vi "1 - 测试基台交互.vi"(6 "测试机台选择":tag="VB8012-30F490B", 8 "逻辑分析仪参数输入":T2, 9 "可编程电源参数输入":T3, 10 "显示控件引用输入":T1) -> (0 "error out":errorcluster caption="错误输出", 2 "采集信号输出":waveform(dbl)[](array[waveform]), 3 "显示控件引用输出":T1)   [LabVIEW 2019]
uses:
  <vilib>/VirtualBench/_PS Configure Voltage Output0.vi
  <vilib>/VirtualBench/_FGEN Configure Standard Waveform14.vi
  <vilib>/VirtualBench/_MSO Configure Timing0.vi
  <vilib>/VirtualBench/_MSO Configure Digital Edge Trigger0.vi
  <vilib>/VirtualBench/_MSO Configure Analog Edge Trigger0.vi
  <vilib>/VirtualBench/_MSO Configure Digital Pattern Trigger0.vi
  <vilib>/VirtualBench/_FGEN Configure Standard Waveform0.vi
  <vilib>/VirtualBench/VirtualBench.lvlib
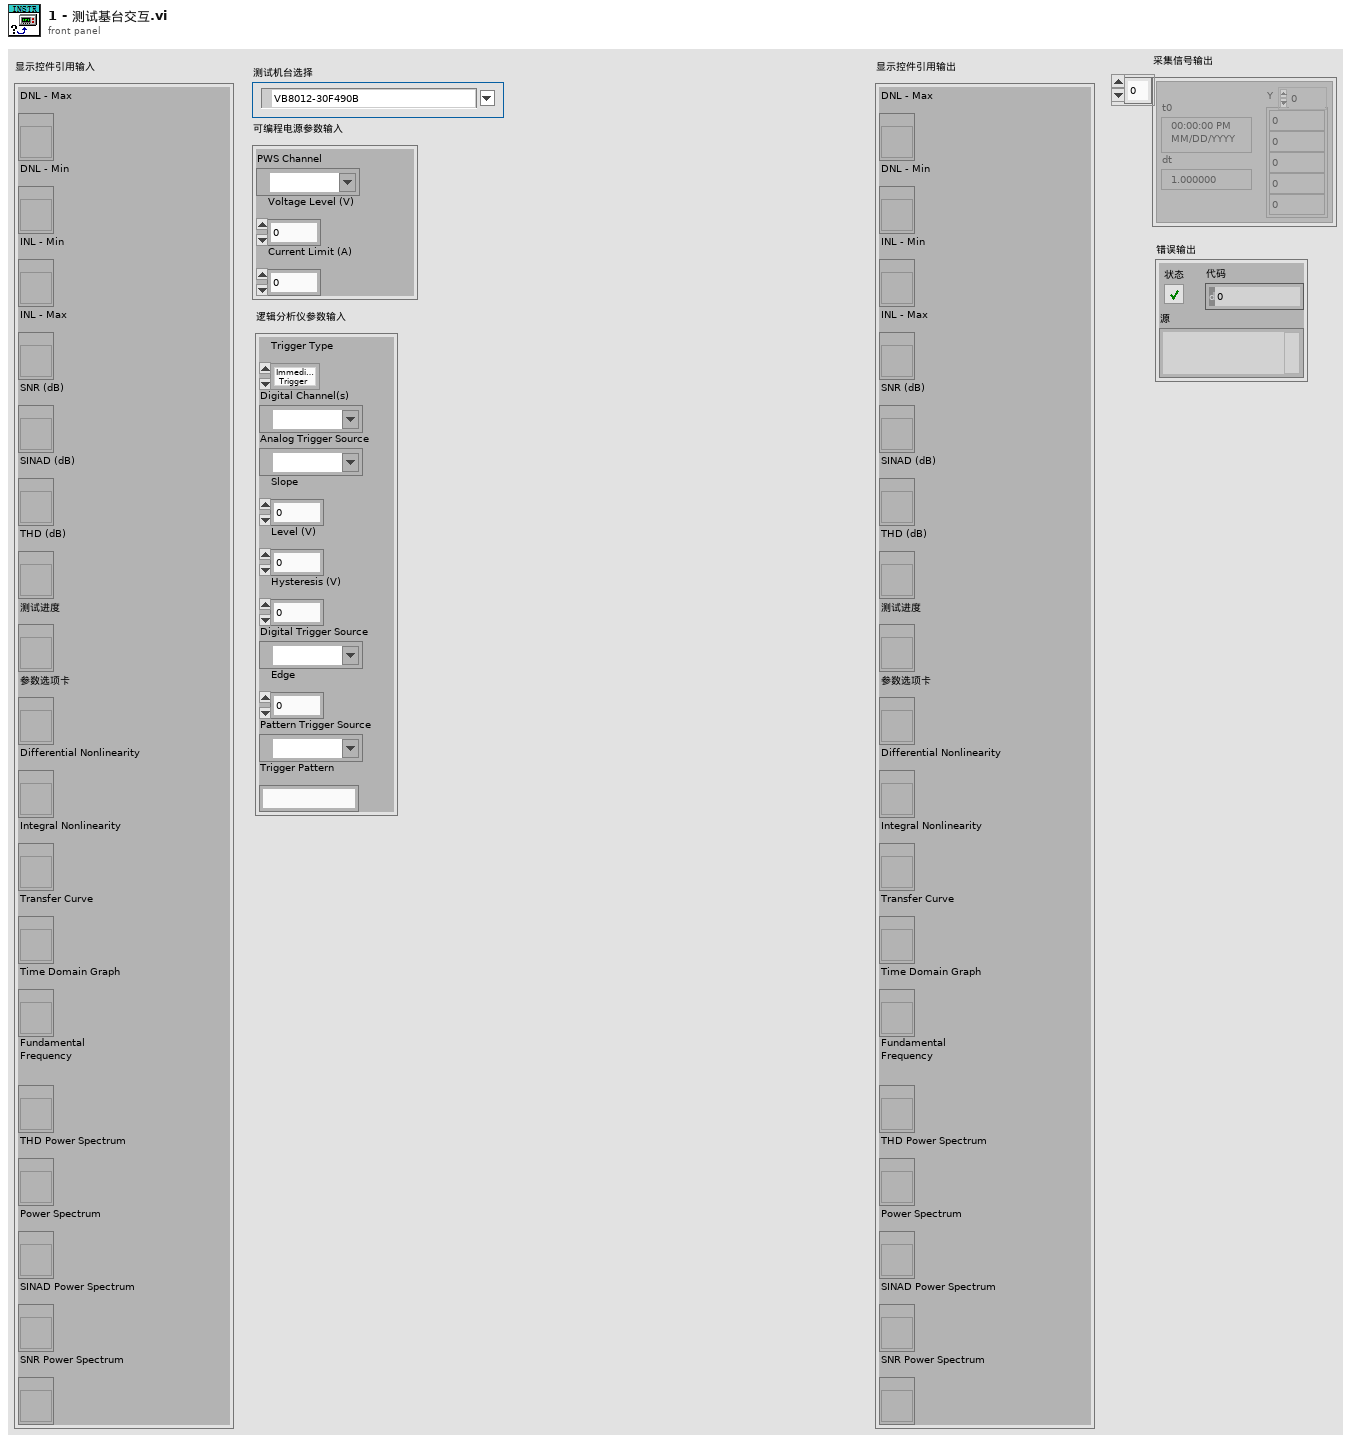
[diagram p1: front panel]
types:
  T1 = cluster{"DNL - Max":refnum<vi>, "DNL - Min":refnum<vi>, "INL - Min":refnum<vi>, "INL - Max":refnum<vi>, "SNR (dB)":refnum<vi>, "SINAD (dB)":refnum<vi>, "THD (dB)":refnum<vi>, "测试进度":refnum<vi>, "参数选项卡":refnum<vi>, "Differential Nonlinearity":refnum<vi>, "Integral Nonlinearity":refnum<vi>, "Transfer Curve":refnum<vi>, "Time Domain Graph":refnum<vi>, "Fundamental\nFrequency":refnum<vi>, "THD Power Spectrum":refnum<vi>, "Power Spectrum":refnum<vi>, "SINAD Power Spectrum":refnum<vi>, "SNR Power Spectrum":refnum<vi>}
  T2 = cluster{"Trigger Type":enum32{"Immediate Trigger", "Digital Trigger", "Analog Trigger", "Pattern Trigger"}, "Digital Channel(s)":tag, "Analog Trigger Source":tag, "Slope":i32, "Level (V)":dbl, "Hysteresis (V)":dbl, "Digital Trigger Source":tag, "Edge":i32, "Pattern Trigger Source":tag, "Trigger Pattern":string}
  T3 = cluster{"PWS Channel":tag, "Voltage Level (V)":dbl, "Current Limit (A)":dbl}
  T4 = enum32{"Time Domain", "Power Spectrum", "THD", "SINAD", "SNR", "DNL", "INL", "Transfer Curve"}
  T5 = enum32{"Immediate Trigger", "Digital Trigger", "Analog Trigger", "Pattern Trigger"}
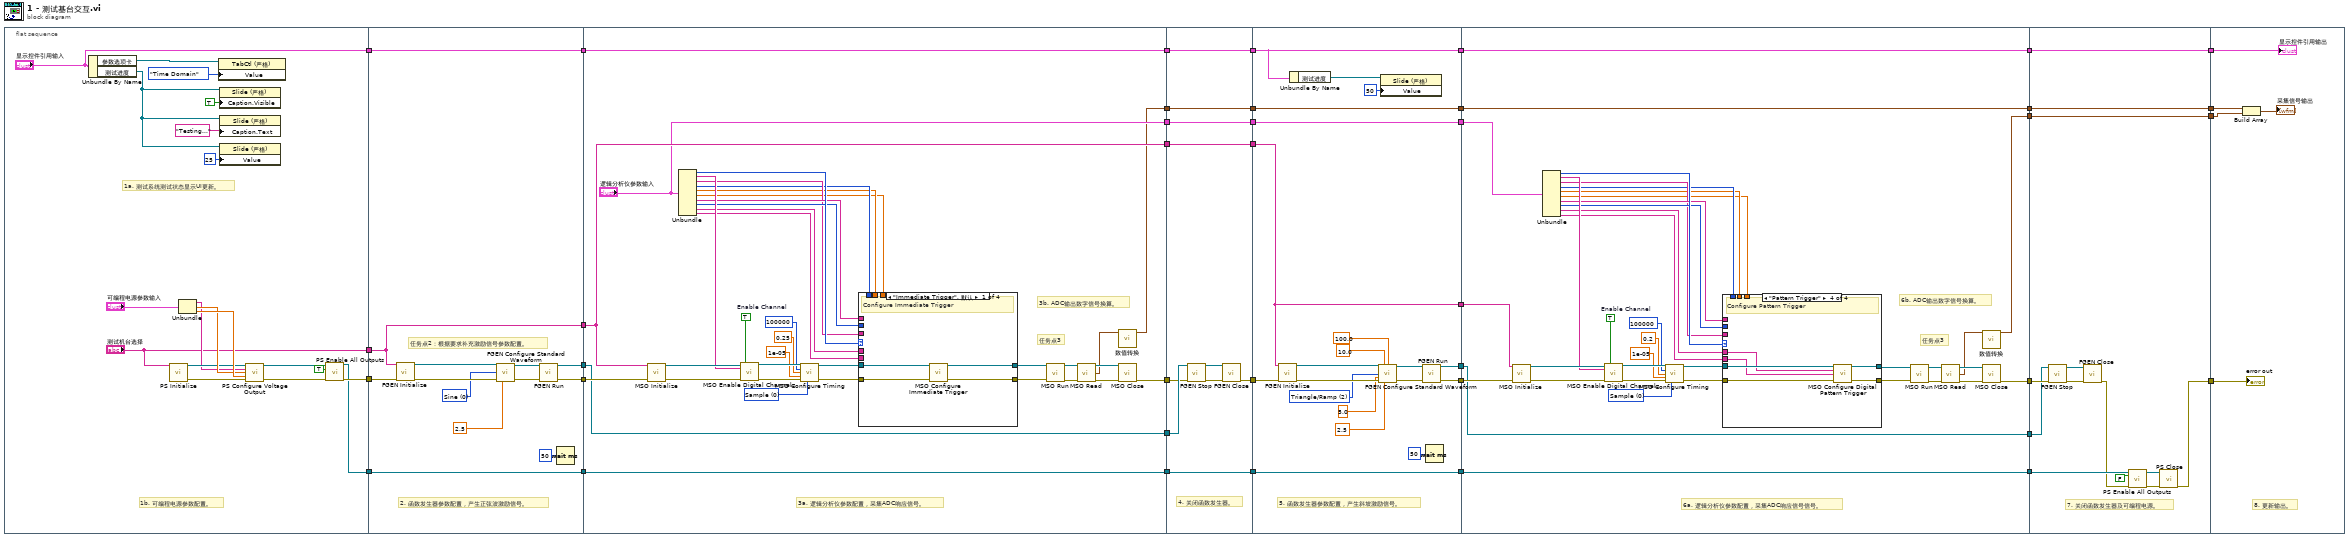
[diagram p0: block diagram]
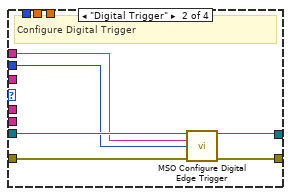
[diagram p2: hidden frame]
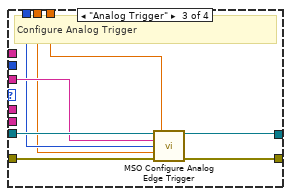
[diagram p3: hidden frame]
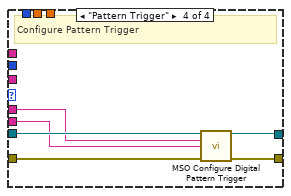
[diagram p4: hidden frame]
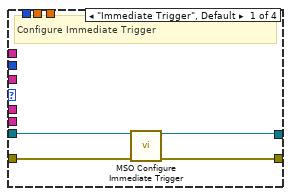
[diagram p5: hidden frame]
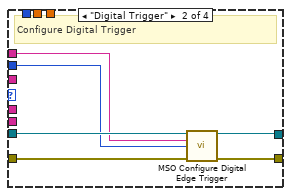
[diagram p6: hidden frame]
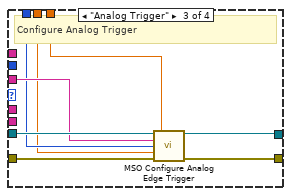
[diagram p7: hidden frame]
diagram:
  n1 = flat-sequence {
    tunnel: [w49] -> w39
    tunnel: ["测试机台选择"] -> w38
    tunnel: ["显示控件引用输入"] -> w8
    tunnel: [w47] -> w6
    tunnel: w39 -> [w67]
    tunnel: w38 -> [w62]
    tunnel: [w64] -> w37
    tunnel: [w63] -> w36
    tunnel: [w62] -> w35
    tunnel: [w61] -> w9
    tunnel: w8 -> [w61]
    tunnel: w6 -> [w60]
    tunnel: [w60] -> w1
    tunnel: w37 -> [w78]
    tunnel: w36 -> [w95]
    tunnel: w35 -> [w76]
    tunnel: [w78] -> w34
    tunnel: [w77] -> w33
    tunnel: [w76] -> w30
    tunnel: ["逻辑分析仪参数输入"] -> w25
    tunnel: [w74] -> w21
    tunnel: [w73] -> w10
    tunnel: w9 -> [w73]
    tunnel: [w72] -> w2
    tunnel: w1 -> [w72]
    tunnel: w34 -> [w140]
    tunnel: w33 -> [w139]
    tunnel: [w137] -> w32
    tunnel: [w136] -> w31
    tunnel: w30 -> [w136]
    tunnel: [w135] -> w26
    tunnel: w25 -> [w135]
    tunnel: w21 -> [w134]
    tunnel: [w134] -> w18
    tunnel: [w133] -> w11
    tunnel: w10 -> [w133]
    tunnel: [w132] -> w3
    tunnel: w2 -> [w132]
    tunnel: w32 -> [w152]
    tunnel: w31 -> [w149]
    tunnel: [w151] -> w29
    tunnel: [w150] -> w28
    tunnel: [w149] -> w27
    tunnel: w26 -> [w148]
    tunnel: [w148] -> w24
    tunnel: [w147] -> w19
    tunnel: w18 -> [w147]
    tunnel: [w142] -> w12
    tunnel: w11 -> [w142]
    tunnel: [w146] -> w4
    tunnel: w3 -> [w146]
    tunnel: w29 -> [w171]
    tunnel: w28 -> [w167]
    tunnel: w27 -> [w170]
    tunnel: w24 -> [w169]
    tunnel: [w168] -> w23
    tunnel: [w167] -> w22
    tunnel: [w166] -> w20
    tunnel: w19 -> [w166]
    tunnel: [w163] -> w17
    tunnel: [w165] -> w13
    tunnel: w12 -> [w165]
    tunnel: [w164] -> w5
    tunnel: w4 -> [w164]
    tunnel: w23 -> [w233]
    tunnel: w22 -> [w232]
    tunnel: w20 -> [w231]
    tunnel: w17 -> [w230]
    tunnel: [w231] -> w16
    tunnel: [w230] -> w15
    tunnel: [w229] -> w14
    tunnel: w13 -> [w229]
    tunnel: [w223] -> w7
    tunnel: w5 -> [w225]
    tunnel: w16 -> [w240]
    tunnel: w15 -> [w239]
    tunnel: w14 -> [w236]
    tunnel: w7 -> [w237]
    frame #0 {
      # "1b. 可编程电源参数配置。"
      # "1a. 测试系统测试状态显示UI更新。"
      n2 = Unbundle By Name("显示控件引用输入") -> ("参数选项卡"=w46:refnum<vi>, "测试进度"=w42:refnum<vi>)
      n3 = call <vilib>:"PS Initialize.vi"("Device Name"="测试机台选择") -> ("Instrument Handle Out"=w55:refnum<k21>, "Error Out"=w51:errorcluster)  [unwired: 13 in]
      n4 = Unbundle("可编程电源参数输入") -> ("PWS Channel"=w54:tag, "Voltage Level (V)"=w56:dbl, "Current Limit (A)"=w57:dbl)
      n5 = property class="TabCtl (严格)"(reference=w46, "Value"=T4."Time Domain" ("值")) -> ()  [unwired: 1 in, 2 out]
      n6 = property class="Slide (严格)"(reference=w42, "Caption.Visible"=TRUE ("标题.可见")) -> ()  [unwired: 1 in, 2 out]
      n7 = property class="Slide (严格)"(reference=w42, "Caption.Text"="Testing..." ("标题.文本")) -> ()  [unwired: 1 in, 2 out]
      n8 = property class="Slide (严格)"(reference=w42, "Value"=u8 25 ("值")) -> ()  [unwired: 1 in, 2 out]
      n9 = call-poly <vilib>:"PS Configure Voltage Output.vi"("Instrument Handle In"=w55, "Channel"=w54, "Voltage Level"=w56, "Current Limit"=w57, "Error In"=w51) -> ("Instrument Handle Out"=w58:refnum<k21>, "Error Out"=w52:errorcluster)  [unwired: 9 in]
      n10 = call <vilib>:"PS Enable All Outputs.vi"("Instrument Handle In"=w58, "Enable Outputs"=TRUE ("Enable Output"), "Error In"=w52) -> ("Instrument Handle Out"=w47:refnum<k21>, "Error Out"=w49:errorcluster)  [unwired: 11 in]
    }
    frame #1 {
      w66 = 0 items=["Sine", "Square", "Triangle/Ramp", "DC"] ("Waveform Function")
      # "任务点2：根据要求补充激励信号参数配置。"
      # "2. 函数发生器参数配置，产生正弦波激励信号。"
      n11 = call <vilib>:"FGEN Initialize.vi"("Device Name"=w62, "Error In"=w67) -> ("Instrument Handle Out"=w68:refnum<k21>, "Error Out"=w69:errorcluster)  [unwired: 12 in]
      n12 = call-poly <vilib>:"FGEN Configure Standard Waveform.vi"("Instrument Handle In"=w68, "Waveform Function"=w66, "Error In"=w69, "DC Offset"=2.5 ("DC Offset (V)")) -> ("Instrument Handle Out"=w70:refnum<k21>, "Error Out"=w71:errorcluster)  [unwired: 10 in]
      n13 = call <vilib>:"FGEN Run.vi"("Instrument Handle In"=w70, "Error In"=w71) -> ("Instrument Handle Out"=w64:refnum<k21>, "Error Out"=w63:errorcluster)  [unwired: 12 in]
      n14 = Wait (ms)(milliseconds to wait=u32 50 ("等待时间（毫秒）")) -> ()  [unwired: 1 out]
    }
    frame #2 {
      w102 = TRUE  # Enable Channel
      w107 = 0 items=["Sample", "Peak Detect"] ("Sampling Mode")
      # "任务点3"
      # "3b. ADC输出数字信号换算。"
      # "3a. 逻辑分析仪参数配置，采集ADC响应信号。"
      n15 = call <vilib>:"MSO Initialize.vi"("Device Name"=w76, "Error In"=w95) -> ("Instrument Handle Out"=w99:refnum<k21>, "Error Out"=w98:errorcluster)  [unwired: 12 in]
      n16 = Unbundle("逻辑分析仪参数输入") -> ("Trigger Type"=w90:T5, "Digital Channel(s)"=w94:tag, "Analog Trigger Source"=w87:tag, "Slope"=w86:i32, "Level (V)"=w85:dbl, "Hysteresis (V)"=w84:dbl, "Digital Trigger Source"=w89:tag, "Edge"=w88:i32, "Pattern Trigger Source"=w83:tag, "Trigger Pattern"=w82:string)
      n17 = call <vilib>:"MSO Enable Digital Channels.vi"("Instrument Handle In"=w99, "Enable Channel"=w102, "Channel"=w94, "Error In"=w98) -> ("Instrument Handle Out"=w103:refnum<k21>, "Error Out"=w104:errorcluster)  [unwired: 10 in]
      n18 = call-poly <vilib>:"MSO Configure Timing.vi"("Instrument Handle In"=w103, "Sample Rate"=100000 ("Sample Rate (Hz)"), "Acquisition Time (s)"=0.25, "Pretrigger Time (s)"=1e-05, "Error In"=w104, "Sampling Mode"=w107) -> ("Instrument Handle Out"=w106:refnum<k21>, "Error Out"=w105:errorcluster)  [unwired: 8 in]
      n19 = case shown="\"Immediate Trigger\", 默认" w90 {
        tunnel: w106 -> [w111 w115 w122 w129]
        tunnel: w105 -> [w109 w116 w125 w128]
        tunnel: [w110 w114 w123 w130] -> w97
        tunnel: [w108 w117 w124 w131] -> w96
        tunnel: w89 -> [_ w113 _ _]
        tunnel: w88 -> [_ w112 _ _]
        tunnel: w87 -> [_ _ w121 _]
        tunnel: w86 -> [_ _ w120 _]
        tunnel: w85 -> [_ _ w119 _]
        tunnel: w84 -> [_ _ w118 _]
        tunnel: w83 -> [_ _ _ w127]
        tunnel: w82 -> [_ _ _ w126]
        frame "Immediate Trigger", Default {
          # "Configure Immediate Trigger"
          n20 = call <vilib>:"MSO Configure Immediate Trigger.vi"("Instrument Handle In"=w111, "Error In"=w109) -> ("Instrument Handle Out"=w110:refnum<k21>, "Error Out"=w108:errorcluster)  [unwired: 12 in]
        }
        frame "Digital Trigger" {
          # "Configure Digital Trigger"
          n21 = call-poly <vilib>:"MSO Configure Digital Edge Trigger.vi"("Instrument Handle In"=w115, "Trigger Source"=w113, "Trigger Slope"=w112, "Error In"=w116) -> ("Instrument Handle Out"=w114:refnum<k21>, "Error Out"=w117:errorcluster)  [unwired: 10 in]
        }
        frame "Analog Trigger" {
          # "Configure Analog Trigger"
          n22 = call-poly <vilib>:"MSO Configure Analog Edge Trigger.vi"("Instrument Handle In"=w122, "Trigger Hysteresis"=w118, "Trigger Source"=w121, "Trigger Slope"=w120, "Trigger Level"=w119, "Error In"=w125) -> ("Instrument Handle Out"=w123:refnum<k21>, "Error Out"=w124:errorcluster)  [unwired: 8 in]
        }
        frame "Pattern Trigger" {
          # "Configure Pattern Trigger"
          n23 = call-poly <vilib>:"MSO Configure Digital Pattern Trigger.vi"("Instrument Handle In"=w129, "Trigger Source"=w127, "Trigger Pattern"=w126, "Error In"=w128) -> ("Instrument Handle Out"=w130:refnum<k21>, "Error Out"=w131:errorcluster)  [unwired: 10 in]
        }
      }
      n24 = call <vilib>:"MSO Run.vi"("Instrument Handle In"=w97, "Error In"=w96) -> ("Instrument Handle Out"=w101:refnum<k21>, "Error Out"=w100:errorcluster)  [unwired: 12 in]
      n25 = call <vilib>:"MSO Read.vi"("Instrument Handle In"=w101, "Error In"=w100) -> ("Instrument Handle Out"=w80:refnum<k21>, "Digital Waveform"=w79:digitalwaveform, "Error Out"=w81:errorcluster)  [unwired: 8 in, 3 out]
      n26 = call "数值转换.vi"("Digital Waveform"=w79) -> ("Waveform"=w74:waveform(dbl))  [unwired: 9 in, 1 out]
      n27 = call <vilib>:"MSO Close.vi"("Instrument Handle In"=w80, "Error In"=w81) -> ("Error Out"=w77:errorcluster)  [unwired: 13 in]
    }
    frame #3 {
      # "4. 关闭函数发生器。"
      n28 = call <vilib>:"FGEN Stop.vi"("Instrument Handle In"=w140, "Error In"=w139) -> ("Instrument Handle Out"=w138:refnum<k21>, "Error Out"=w141:errorcluster)  [unwired: 12 in]
      n29 = call <vilib>:"FGEN Close.vi"("Instrument Handle In"=w138, "Error In"=w141) -> ("Error Out"=w137:errorcluster)  [unwired: 13 in]
    }
    frame #4 {
      w155 = 2 items=["Sine", "Square", "Triangle/Ramp", "DC"] ("Waveform Function")
      # "5. 函数发生器参数配置，产生斜坡激励信号。"
      n30 = call <vilib>:"FGEN Initialize.vi"("Device Name"=w149, "Error In"=w152) -> ("Instrument Handle Out"=w158:refnum<k21>, "Error Out"=w159:errorcluster)  [unwired: 12 in]
      n31 = Unbundle By Name(w142) -> ("测试进度"=w144:refnum<vi>)
      n32 = call-poly <vilib>:"FGEN Configure Standard Waveform.vi"("Instrument Handle In"=w158, "Frequency"=10.0 ("Frequency (Hz)"), "Duty Cycle"=100.0, "Waveform Function"=w155, "Amplitude"=5.0 ("Amplitude (V)"), "Error In"=w159, "DC Offset"=2.5 ("DC Offset (V)")) -> ("Instrument Handle Out"=w160:refnum<k21>, "Error Out"=w161:errorcluster)  [unwired: 7 in]
      n33 = property class="Slide (严格)"(reference=w144, "Value"=u8 50 ("值")) -> ()  [unwired: 1 in, 2 out]
      n34 = call <vilib>:"FGEN Run.vi"("Instrument Handle In"=w160, "Error In"=w161) -> ("Instrument Handle Out"=w150:refnum<k21>, "Error Out"=w151:errorcluster)  [unwired: 12 in]
      n35 = Wait (ms)(milliseconds to wait=u32 50 ("等待时间（毫秒）")) -> ()  [unwired: 1 out]
    }
    frame #5 {
      w193 = TRUE  # Enable Channel
      w198 = 0 items=["Sample", "Peak Detect"] ("Sampling Mode")
      # "任务点3"
      # "6b. ADC输出数字信号换算。"
      # "6a. 逻辑分析仪参数配置，采集ADC响应信号信号。"
      n36 = call <vilib>:"MSO Initialize.vi"("Device Name"=w170, "Error In"=w171) -> ("Instrument Handle Out"=w190:refnum<k21>, "Error Out"=w189:errorcluster)  [unwired: 12 in]
      n37 = Unbundle(w169) -> ("Trigger Type"=w182:T5, "Digital Channel(s)"=w186:tag, "Analog Trigger Source"=w179:tag, "Slope"=w178:i32, "Level (V)"=w177:dbl, "Hysteresis (V)"=w176:dbl, "Digital Trigger Source"=w181:tag, "Edge"=w180:i32, "Pattern Trigger Source"=w175:tag, "Trigger Pattern"=w174:string)
      n38 = call <vilib>:"MSO Enable Digital Channels.vi"("Instrument Handle In"=w190, "Enable Channel"=w193, "Channel"=w186, "Error In"=w189) -> ("Instrument Handle Out"=w194:refnum<k21>, "Error Out"=w195:errorcluster)  [unwired: 10 in]
      n39 = call-poly <vilib>:"MSO Configure Timing.vi"("Instrument Handle In"=w194, "Sample Rate"=100000 ("Sample Rate (Hz)"), "Acquisition Time (s)"=0.2, "Pretrigger Time (s)"=1e-05, "Error In"=w195, "Sampling Mode"=w198) -> ("Instrument Handle Out"=w197:refnum<k21>, "Error Out"=w196:errorcluster)  [unwired: 8 in]
      n40 = case shown="\"Pattern Trigger\"" w182 {
        tunnel: w197 -> [w202 w206 w213 w220]
        tunnel: w196 -> [w200 w207 w216 w219]
        tunnel: [w201 w205 w214 w221] -> w188
        tunnel: [w199 w208 w215 w222] -> w187
        tunnel: w181 -> [_ w204 _ _]
        tunnel: w180 -> [_ w203 _ _]
        tunnel: w179 -> [_ _ w212 _]
        tunnel: w178 -> [_ _ w211 _]
        tunnel: w177 -> [_ _ w210 _]
        tunnel: w176 -> [_ _ w209 _]
        tunnel: w175 -> [_ _ _ w218]
        tunnel: w174 -> [_ _ _ w217]
        frame "Immediate Trigger", Default {
          # "Configure Immediate Trigger"
          n41 = call <vilib>:"MSO Configure Immediate Trigger.vi"("Instrument Handle In"=w202, "Error In"=w200) -> ("Instrument Handle Out"=w201:refnum<k21>, "Error Out"=w199:errorcluster)  [unwired: 12 in]
        }
        frame "Digital Trigger" {
          # "Configure Digital Trigger"
          n42 = call-poly <vilib>:"MSO Configure Digital Edge Trigger.vi"("Instrument Handle In"=w206, "Trigger Source"=w204, "Trigger Slope"=w203, "Error In"=w207) -> ("Instrument Handle Out"=w205:refnum<k21>, "Error Out"=w208:errorcluster)  [unwired: 10 in]
        }
        frame "Analog Trigger" {
          # "Configure Analog Trigger"
          n43 = call-poly <vilib>:"MSO Configure Analog Edge Trigger.vi"("Instrument Handle In"=w213, "Trigger Hysteresis"=w209, "Trigger Source"=w212, "Trigger Slope"=w211, "Trigger Level"=w210, "Error In"=w216) -> ("Instrument Handle Out"=w214:refnum<k21>, "Error Out"=w215:errorcluster)  [unwired: 8 in]
        }
        frame "Pattern Trigger" {
          # "Configure Pattern Trigger"
          n44 = call-poly <vilib>:"MSO Configure Digital Pattern Trigger.vi"("Instrument Handle In"=w220, "Trigger Source"=w218, "Trigger Pattern"=w217, "Error In"=w219) -> ("Instrument Handle Out"=w221:refnum<k21>, "Error Out"=w222:errorcluster)  [unwired: 10 in]
        }
      }
      n45 = call <vilib>:"MSO Run.vi"("Instrument Handle In"=w188, "Error In"=w187) -> ("Instrument Handle Out"=w192:refnum<k21>, "Error Out"=w191:errorcluster)  [unwired: 12 in]
      n46 = call <vilib>:"MSO Read.vi"("Instrument Handle In"=w192, "Error In"=w191) -> ("Instrument Handle Out"=w172:refnum<k21>, "Digital Waveform"=w162:digitalwaveform, "Error Out"=w173:errorcluster)  [unwired: 8 in, 3 out]
      n47 = call "数值转换.vi"("Digital Waveform"=w162) -> ("Waveform"=w163:waveform(dbl))  [unwired: 9 in, 1 out]
      n48 = call <vilib>:"MSO Close.vi"("Instrument Handle In"=w172, "Error In"=w173) -> ("Error Out"=w168:errorcluster)  [unwired: 13 in]
    }
    frame #6 {
      # "7. 关闭函数发生器及可编程电源。"
      n49 = call <vilib>:"FGEN Stop.vi"("Instrument Handle In"=w232, "Error In"=w233) -> ("Instrument Handle Out"=w235:refnum<k21>, "Error Out"=w234:errorcluster)  [unwired: 12 in]
      n50 = call <vilib>:"FGEN Close.vi"("Instrument Handle In"=w235, "Error In"=w234) -> ("Error Out"=w224:errorcluster)  [unwired: 13 in]
      n51 = call <vilib>:"PS Enable All Outputs.vi"("Instrument Handle In"=w225, "Enable Outputs"=FALSE ("Enable Output"), "Error In"=w224) -> ("Instrument Handle Out"=w228:refnum<k21>, "Error Out"=w227:errorcluster)  [unwired: 11 in]
      n52 = call <vilib>:"PS Close.vi"("Instrument Handle In"=w228, "Error In"=w227) -> ("Error Out"=w223:errorcluster)  [unwired: 13 in]
    }
    frame #7 {
      # "8. 更新输出。"
      n53 = Build Array(w240, w239) -> (→"采集信号输出":waveform(dbl)[])
      "error out" <- w237
      "显示控件引用输出" <- w236
    }
  }
